vi "Discover Available Cameras.vi"(8 "error in (no error)":errorcluster, 11 "TLCameraSDK reference":refnum<k24>) -> (0 "error out":errorcluster, 1 "Serial Numbers":string[](array[string]), 2 "Number of Cameras":i32, 3 "TLCameraSDK reference out":refnum<k24>)   [LabVIEW 2020]
uses:
  C:/GEECS/Developers Version/builds/Device builds/ThorlabsCsCamera/Thorlabs.TSI.TLCameraInterfaces.dll
  Thorlabs.TSI.TLCameraInterfaces.dll
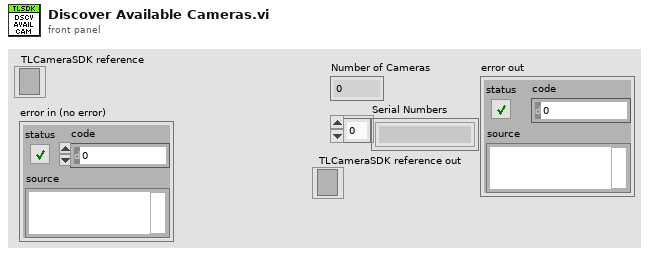
[diagram p1: front panel]
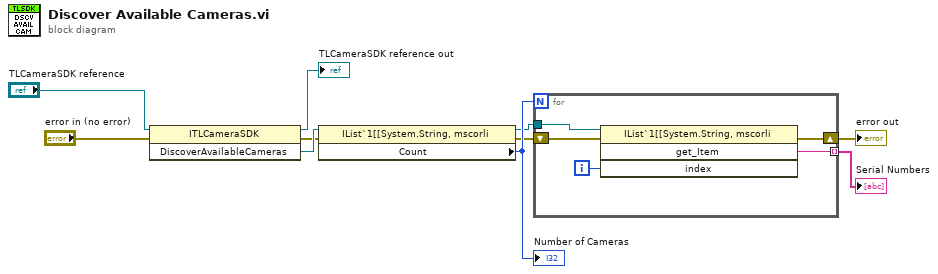
[diagram p0: block diagram]
diagram:
  n1 = invoke class="ITLCameraSDK" method="DiscoverAvailableCameras"(reference="TLCameraSDK reference", error in="error in (no error)") -> (reference out=→"TLCameraSDK reference out":refnum<k24>, error out=w8:errorcluster, "DiscoverAvailableCameras"=w10:refnum<k24>)  [unwired: 1 in]
  n2 = property class="IList`1[[System.String, mscorli"(reference=w10, error in=w8) -> (reference out=w6:refnum<k24>, error out=w5:errorcluster, "Count"=w7:i32)
  "Number of Cameras" <- w7
  n3 = for {
    N: w7 -> [_]
    tunnel: w6 -> [w15]
    shift-right: [w13] -> w2
    shift-left: w5 -> [w14]
    tunnel: [w11] -> w4 mode=indexing
    i -> [w12]
    n4 = invoke class="IList`1[[System.String, mscorli" method="get_Item"(reference=w15, error in=w14, "index"=w12) -> (error out=w13:errorcluster, "get_Item"=w11:string)  [unwired: 1 in, 2 out]
  }
  "Serial Numbers" <- w4
  "error out" <- w2
